vi "Check if linker vi is under vilib.vi"(10 "Include VI.lib":bool, 11 "path":path) -> (3 "Include Info":bool)   [LabVIEW 2019, in "SimpleDependencyInspector.lvlib"]
uses:
  SimpleDependencyInspector.lvlib
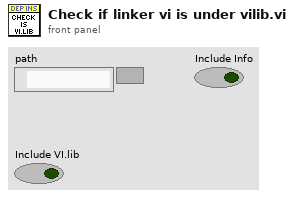
[diagram p1: front panel]
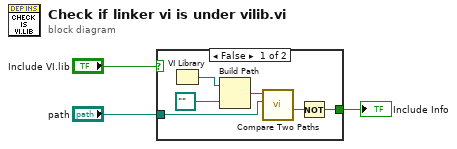
[diagram p0: block diagram]
diagram:
  n1 = case shown="False" "Include VI.lib" {
    selector: "Include VI.lib" -> [_ w10]
    tunnel: [w6 w10] -> w3
    tunnel: "path" -> [w8 _]
    frame False {
      n2 = VI Library() -> (path=w7:path)
      n3 = Build Path(base path=w7, name or relative path=path "..") -> (appended path=w5:path)
      n4 = call <vilib>:"Compare Two Paths.vi"("Path 2"=w8, "Path 1"=w5) -> ("Path 2 Relative to Path 1?"=w9:bool)  [unwired: 6 in, 3 out]
      n5 = Not(x=w9) -> (.not. x?=w6:bool)
    }
    frame True {
    }
  }
  "Include Info" <- w3
